vi "cmdConnectDB.vi"(1 "input_bool_local":bool=TRUE) -> (0 "show_str_state":string)   [LabVIEW 2011]
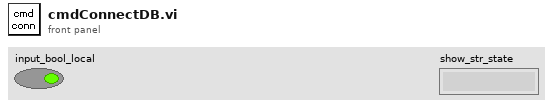
[diagram p1: front panel]
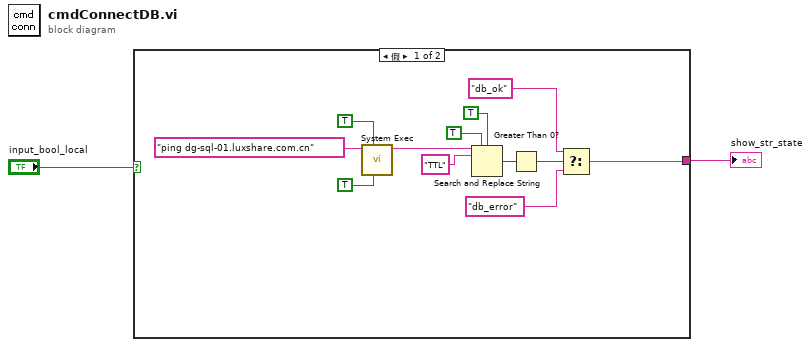
[diagram p0: block diagram]
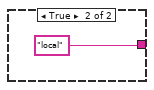
[diagram p2: hidden frame]
diagram:
  n1 = case shown="假" "input_bool_local" {
    tunnel: [w8 "local"] -> w1
    frame False {
      n2 = call <vilib>:"System Exec.vi"("run minimized? (F)"=TRUE, "wait until completion? (T)"=TRUE, "command line"="ping dg-sql-01.luxshare.com.cn") -> ("standard output"=w4:string)  [unwired: 5 in, 3 out]
      n3 = Search and Replace String(replace all?=TRUE ("替换全部？(F)"), case sensitive?=TRUE ("忽略大小写？(F)"), input string=w4, search string="TTL" ("搜索字符串")) -> (number of replacements=w10:i32)  [unwired: 4 in, 3 out]
      n4 = Greater Than 0?(x=w10) -> (x > 0?=w9:bool)
      n5 = Select(t="db_ok", s=w9, f="db_error") -> (s? t:f=w8:string)
    }
    frame True {
    }
  }
  "show_str_state" <- w1
